vi "Read Doc Data.vi"(8 "error in (no error)":errorcluster, 11 "LV MDI.lvclass":refnum<class "LV MDI.lvclass">) -> (0 "error out":errorcluster, 2 "Child Window Data":T1, 3 "LV MDI.lvclass":refnum<class "LV MDI.lvclass">)   [LabVIEW 2016, in "LV MDI.lvclass"]
uses:
  LV MDI.lvclass
  Private/Window Data.ctl
  LV MDI.lvclass/LV MDI.ctl
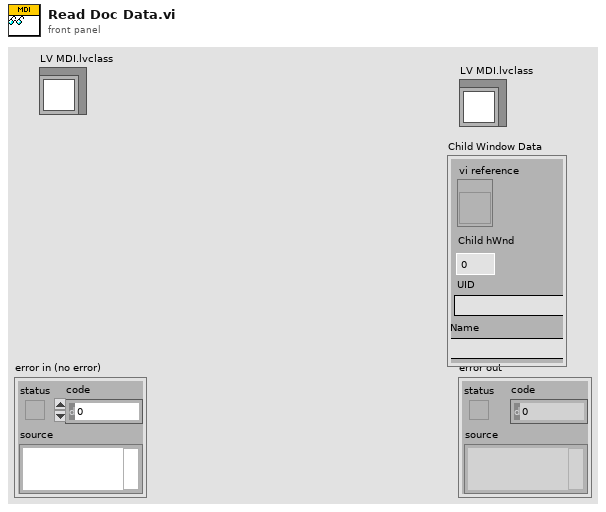
[diagram p1: front panel]
types:
  T1 = typedef "LV MDI.lvclass/Window Data.ctl" = cluster{"Child hWnd":u32, "UID":string, "vi reference":refnum<vi>, "Name":string}
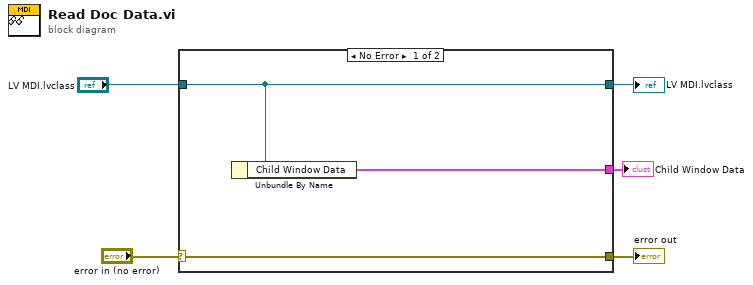
[diagram p0: block diagram]
diagram:
  n1 = case shown="No Error" "error in (no error)" {
    selector: "error in (no error)" -> [w8 w9]
    tunnel: [w8 w9] -> w4
    tunnel: [w7 w10] -> w2
    tunnel: "LV MDI.lvclass" -> [w7 w10]
    tunnel: [w6 _] -> w1
    frame No Error {
      n2 = Unbundle By Name(w7) -> ("Child Window Data"=w6:T1)
    }
    frame Error {
    }
  }
  "error out" <- w4
  "LV MDI.lvclass" <- w2
  "Child Window Data" <- w1
